vi "Msg To.vi"() -> (3 "Pop Up Msg Strategy out":refnum<class "Pop Up Msg Strategy.lvclass">)   [LabVIEW 2021, in "Pop Up.lvlib"]
uses:
  Pop Up.lvlib
  Pop Up Msg Strategy/Pop Up Msg Strategy.lvclass
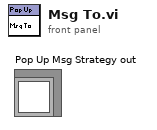
[diagram p1: front panel]
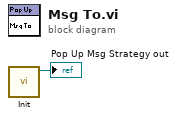
[diagram p0: block diagram]
diagram:
  n1 = call "Init.vi"() -> ("Pop Up Msg Strategy out"=→"Pop Up Msg Strategy out":refnum<class "Pop Up Msg Strategy.lvclass">)  [unwired: 11 in]
